vi "3-Main Combine data.vi"() -> ()   [LabVIEW 2015]
uses:
  <vilib>/Utility/file.llb/Write Delimited Spreadsheet (string).vi
panel:
  in  "Total result path":path=path "I:/2017 Maize-Hyper-Program/2017 Maize Test sample/Result"
  out "8-lg A":path=path "F:/fh/传输D/2015谷粒实验/提取数据/原始总反射率/1-原始总反射率txt"
  out "5-First derivative dA":path=path "F:/fh/传输D/2015谷粒实验/提取数据/原始总反射率/1-原始总反射率txt"
  out "6-Second derivative ddA":path=path "F:/fh/传输D/2015谷粒实验/提取数据/原始总反射率/1-原始总反射率txt"
  out "4-Average reflectance A":path
  out "3-Second derivative ddT":path=path "F:/fh/传输D/2015谷粒实验/提取数据/原始总反射率/1-原始总反射率txt"
  out "2-First derivative dT":path=path "F:/fh/传输D/2015谷粒实验/提取数据/原始总反射率/1-原始总反射率txt"
  out "7-lgT":path=path "F:/fh/传输D/2015谷粒实验/提取数据/原始总反射率/1-原始总反射率txt"
  out "1-Total reflectance T":path=path "F:/fh/传输D/2015谷粒实验/提取数据/原始总反射率/1-原始总反射率txt"
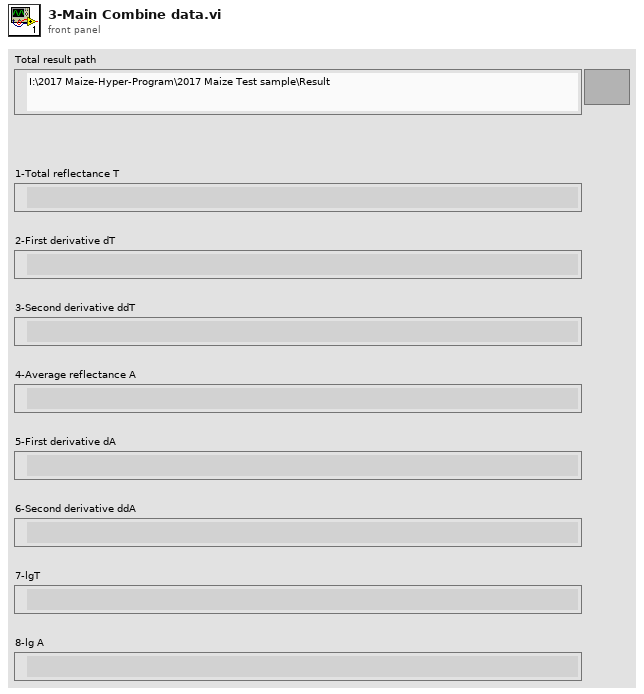
[diagram p1: front panel]
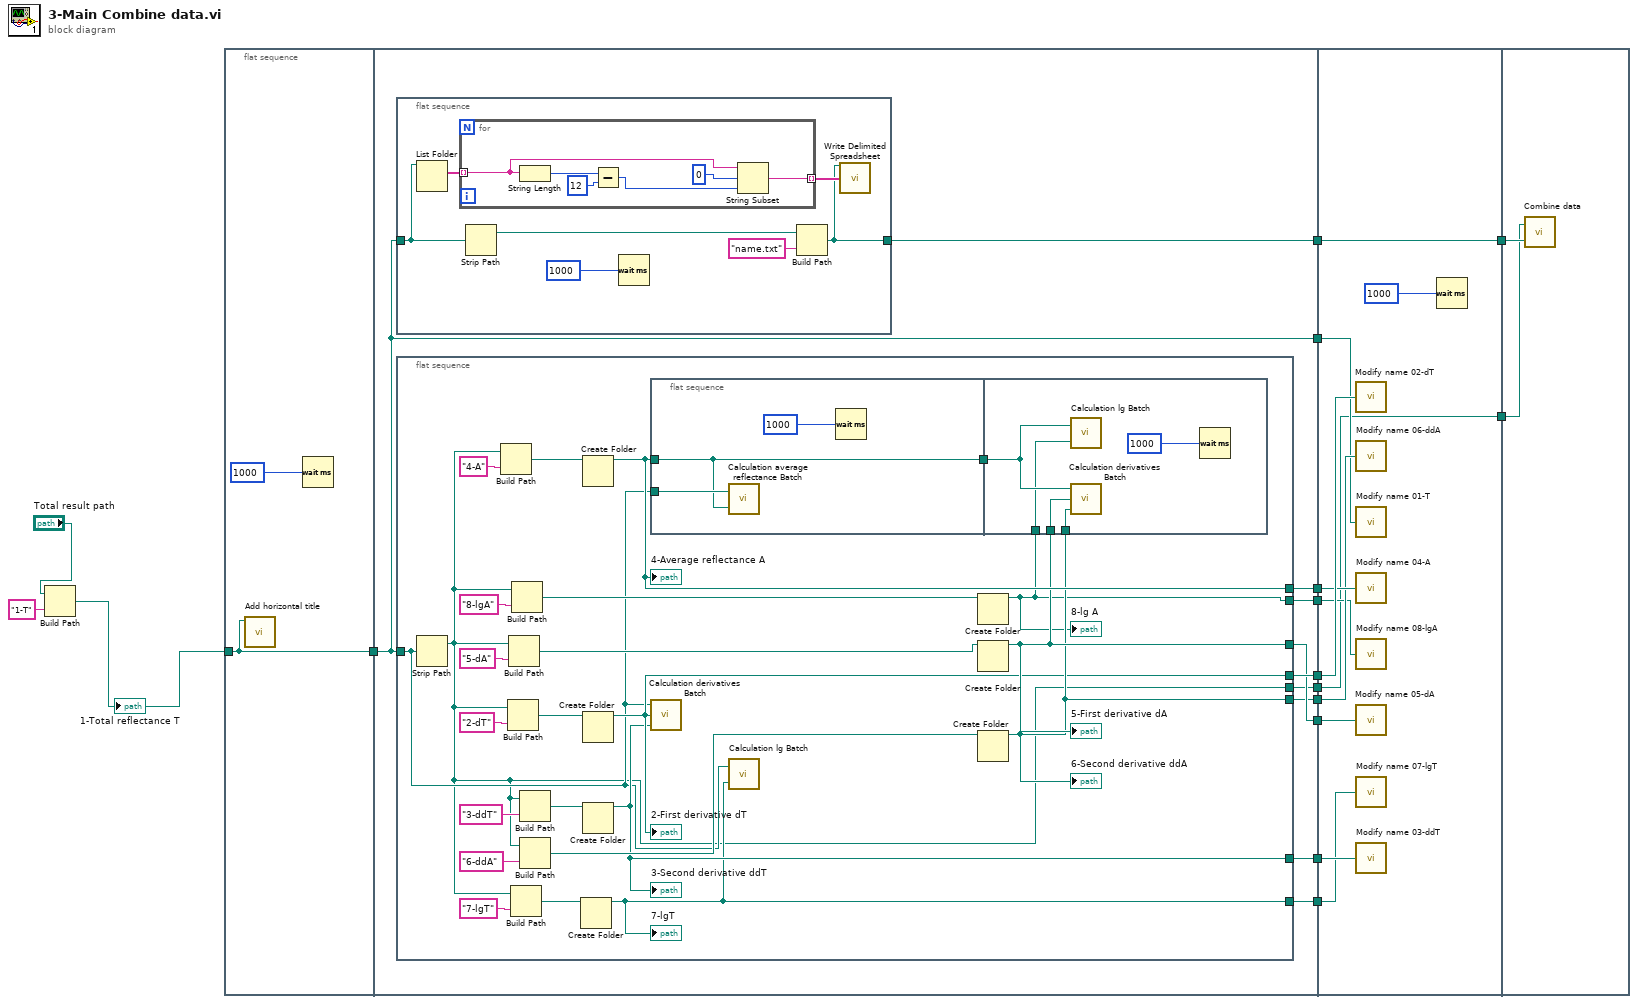
[diagram p0: block diagram]
diagram:
  n1 = Build Path(base path="Total result path", name or relative path="1-T") -> (appended path=w1:path)
  "1-Total reflectance T" <- w1
  n2 = flat-sequence {
    tunnel: w1 -> [w18]
    tunnel: [w18] -> w4
    tunnel: [w28] -> w16
    tunnel: [w27] -> w15
    tunnel: [w26] -> w14
    tunnel: [w25] -> w13
    tunnel: [w24] -> w12
    tunnel: [w23] -> w11
    tunnel: [w22] -> w10
    tunnel: [w21] -> w9
    tunnel: [w20] -> w7
    tunnel: [w19] -> w5
    tunnel: w4 -> [w28]
    tunnel: w16 -> [w76]
    tunnel: w15 -> [w84]
    tunnel: w14 -> [w83]
    tunnel: w13 -> [w82]
    tunnel: w12 -> [w81]
    tunnel: w11 -> [w80]
    tunnel: w10 -> [w79]
    tunnel: w9 -> [w78]
    tunnel: [w77] -> w8
    tunnel: w7 -> [w77]
    tunnel: [w75] -> w6
    tunnel: w5 -> [w75]
    tunnel: w8 -> [w86]
    tunnel: w6 -> [w85]
    frame #0 {
      n3 = call "Add horizontal title.vi"("path"=w18) -> ()  [unwired: 11 in]
      n4 = Wait (ms)(milliseconds to wait=u32 1000 ("millisecond timer value")) -> ()  [unwired: 1 out]
    }
    frame #1 {
      n5 = flat-sequence {
        tunnel: w28 -> [w63]
        tunnel: [w62] -> w20
        frame #0 {
          n6 = List Folder(path=w63) -> (filenames=w64:string[])  [unwired: 3 in, 3 out]
          n7 = for {
            tunnel: w64 -> [w73] mode=indexing
            tunnel: [w68] -> w67 mode=indexing
            n8 = String Length(string=w73) -> (length=w72:i32)
            n9 = Subtract(x=w72, y=12) -> (x-y=w69:i32)
            n10 = String Subset(string=w73, offset (0)=0, length (rest)=w69) -> (substring=w68:string)
          }
          n11 = Strip Path(path=w63) -> (stripped path=w65:path)  [unwired: 1 out]
          n12 = Wait (ms)(milliseconds to wait=u32 1000 ("millisecond timer value")) -> ()  [unwired: 1 out]
          n13 = Build Path(base path=w65, name or relative path="name.txt") -> (appended path=w62:path)
          n14 = call-poly <vilib>:"Write Delimited Spreadsheet.vi"("file path (dialog if empty)"=w62, "1D data"=w67) -> ()  [unwired: 12 in, 2 out]
        }
      }
      n15 = flat-sequence {
        tunnel: w28 -> [w31]
        tunnel: [w33] -> w27
        tunnel: [w32] -> w26
        tunnel: [w37] -> w25
        tunnel: [w36] -> w24
        tunnel: [w35] -> w23
        tunnel: [w30] -> w22
        tunnel: [w34] -> w21
        tunnel: [w29] -> w19
        frame #0 {
          n16 = Strip Path(path=w31) -> (stripped path=w29:path)  [unwired: 1 out]
          n17 = Build Path(base path=w29, name or relative path="4-A") -> (appended path=w46:path)
          n18 = Build Path(base path=w29, name or relative path="2-dT") -> (appended path=w50:path)
          n19 = Build Path(base path=w29, name or relative path="5-dA") -> (appended path=w45:path)
          n20 = Build Path(base path=w29, name or relative path="7-lgT") -> (appended path=w41:path)
          n21 = Build Path(base path=w29, name or relative path="8-lgA") -> (appended path=w38:path)
          n22 = Build Path(base path=w29, name or relative path="3-ddT") -> (appended path=w49:path)
          n23 = Build Path(base path=w29, name or relative path="6-ddA") -> (appended path=w42:path)
          n24 = Create Folder(path (use dialog)=w41) -> (created path=w30:path)  [unwired: 2 in, 2 out]
          "7-lgT" <- w30
          n25 = Create Folder(path (use dialog)=w46) -> (created path=w37:path)  [unwired: 2 in, 2 out]
          "4-Average reflectance A" <- w37
          n26 = Create Folder(path (use dialog)=w50) -> (created path=w33:path)  [unwired: 2 in, 2 out]
          "2-First derivative dT" <- w33
          n27 = Create Folder(path (use dialog)=w49) -> (created path=w32:path)  [unwired: 2 in, 2 out]
          "3-Second derivative ddT" <- w32
          n28 = flat-sequence {
            tunnel: w31 -> [w55]
            tunnel: [w54] -> w52
            tunnel: w37 -> [w54]
            tunnel: w52 -> [w58]
            tunnel: w36 -> [w60]
            tunnel: w35 -> [w59]
            tunnel: w34 -> [w57]
            frame #0 {
              n29 = call "Calculation average reflectance Batch.vi"("保存路径"=w54, "file path (dialog if empty)"=w55) -> ()  [unwired: 1 in]
              n30 = Wait (ms)(milliseconds to wait=u32 1000 ("millisecond timer value")) -> ()  [unwired: 1 out]
            }
            frame #1 {
              n31 = call "Calculation lg Batch.vi"("Savepath"=w57, "file path (dialog if empty)"=w58) -> ()  [unwired: 1 in]
              n32 = call "Calculation derivatives Batch.vi"("Save path 2"=w59, "Save path"=w60, "file path (dialog if empty)"=w58) -> ()  [unwired: 1 in]
              n33 = Wait (ms)(milliseconds to wait=u32 1000 ("millisecond timer value")) -> ()  [unwired: 1 out]
            }
          }
          n34 = call "Calculation derivatives Batch.vi"("Save path 2"=w32, "Save path"=w33, "file path (dialog if empty)"=w31) -> ()  [unwired: 1 in]
          n35 = call "Calculation lg Batch.vi"("Savepath"=w30, "file path (dialog if empty)"=w31) -> ()  [unwired: 1 in]
          n36 = Create Folder(path (use dialog)=w38) -> (created path=w34:path)  [unwired: 2 in, 2 out]
          "8-lg A" <- w34
          n37 = Create Folder(path (use dialog)=w45) -> (created path=w36:path)  [unwired: 2 in, 2 out]
          "5-First derivative dA" <- w36
          n38 = Create Folder(path (use dialog)=w42) -> (created path=w35:path)  [unwired: 2 in, 2 out]
          "6-Second derivative ddA" <- w35
        }
      }
    }
    frame #2 {
      n39 = call "Modify name 02-dT.vi"("path"=w84) -> ()
      n40 = call "Modify name 06-ddA.vi"("path"=w80) -> ()
      n41 = call "Modify name 01-T.vi"("path"=w76) -> ()  [unwired: 1 in]
      n42 = call "Modify name 04-A.vi"("path"=w82) -> ()
      n43 = call "Modify name 08-lgA.vi"("path"=w78) -> ()
      n44 = call "Modify name 05-dA.vi"("path"=w81) -> ()
      n45 = call "Modify name 07-lgT.vi"("path"=w79) -> ()
      n46 = call "Modify name 03-ddT.vi"("path"=w83) -> ()
      n47 = Wait (ms)(milliseconds to wait=u32 1000 ("millisecond timer value")) -> ()  [unwired: 1 out]
    }
    frame #3 {
      n48 = call "Combine data.vi"("name path"=w86, "base path"=w85) -> ()  [unwired: 1 in]
    }
  }
